vi "getEventID.vi"(8 "error in (no error)":errorcluster, 11 "IEventPacket in":refnum<class "IEventPacket.lvclass">) -> (0 "error out":errorcluster, 2 "EventID out":string, 3 "IEventPacket out":refnum<class "IEventPacket.lvclass">)   [LabVIEW 2022 SP3, in "openDAQ.lvlib" / "IBaseObject.lvlib" / "IPacket.lvlib" / "IEventPacket.lvlib" / "IEventPacket.lvclass"]
uses:
  <instrlib>/openDAQ/Public/Classes/IEventPacket/IEventPacket.lvclass
  C:/Program Files (x86)/National Instruments/LabVIEW 2022/instr.lib/openDAQ/Public/Classes/IBaseObject/IBaseObject.lvclass
  <instrlib>/openDAQ/Public/Classes/IBaseObject/IBaseObject.lvclass/IBaseObject.ctl
  <instrlib>/openDAQ/Public/Classes/IBaseObject/Accessor/Read reference.vi
  <instrlib>/openDAQ/Public/Classes/IBaseObject/Accessor/Write reference.vi
  <instrlib>/openDAQ/Public/Classes/daqCoreTypes/IString/IString.lvclass
  <instrlib>/openDAQ/Binaries/Windows/x86/copendaq32.dll
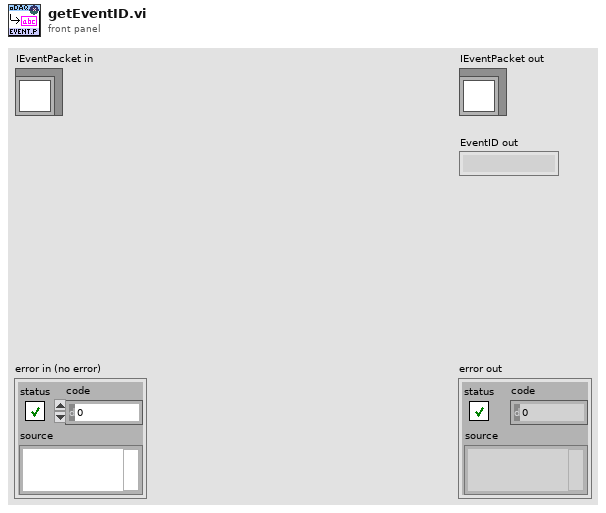
[diagram p1: front panel]
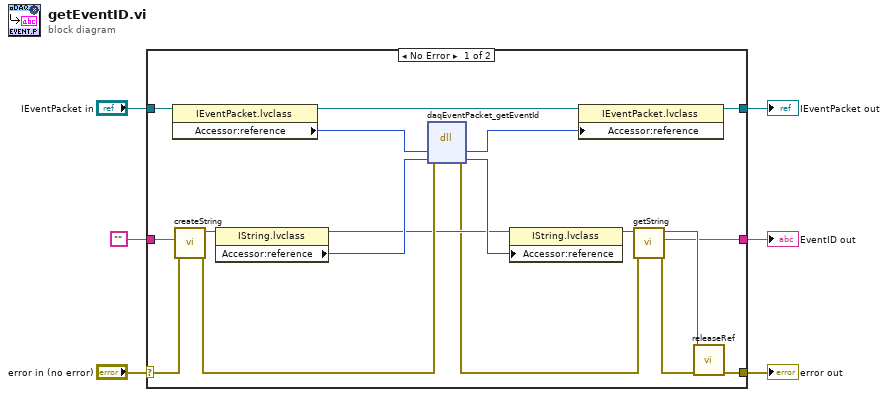
[diagram p0: block diagram]
diagram:
  n1 = case shown="No Error" "error in (no error)" {
    selector: "error in (no error)" -> [w21 w27]
    tunnel: [w12 w27] -> w5
    tunnel: [w7 w26] -> w3
    tunnel: "IEventPacket in" -> [w24 w26]
    tunnel: [w10 w25] -> w1
    tunnel: "" -> [w9 w25]
    frame No Error {
      n2 = property class="IEventPacket.lvclass"(reference=w24) -> (reference out=w8:refnum<class "IEventPacket.lvclass">, "Accessor:reference"=w23:i64)  [unwired: 1 in, 1 out]
      n3 = call <instrlib>:"createString.vi"("error in (no error)"=w21, "String"=w9) -> ("error out"=w20:errorcluster, "IString out"=w19:refnum<class "IString.lvclass">)  [unwired: 8 in]
      n4 = property class="IString.lvclass"(reference=w19) -> (reference out=w16:refnum<class "IString.lvclass">, "Accessor:reference"=w18:i64)  [unwired: 1 in, 1 out]
      n5 = dll-call lib="C:/Program Files (x86)/National Instruments/LabVIEW 2022/instr.lib/openDAQ/Binaries/Windows/x86/copendaq*.*" fn="daqEventPacket_getEventId"(error in=w20, "eventPacket"=w23, "eventId"=w18) -> (error out=w14:errorcluster, "eventPacket"=w22:i64, "eventId"=w17:i64)  [unwired: 3 in, 1 out]
      n6 = property class="IString.lvclass"(reference=w16, "Accessor:reference"=w17) -> (reference out=w15:refnum<class "IString.lvclass">)  [unwired: 1 in, 1 out]
      n7 = property class="IEventPacket.lvclass"(reference=w8, "Accessor:reference"=w22) -> (reference out=w7:refnum<class "IEventPacket.lvclass">)  [unwired: 1 in, 1 out]
      n8 = call <instrlib>:"getString.vi"("error in (no error)"=w14, "IString in"=w15) -> ("error out"=w13:errorcluster, "String out"=w10:string, "IString out"=w11:refnum<class "IString.lvclass">)  [unwired: 7 in]
      n9 = call-dynamic "releaseRef.vi"("error in (no error)"=w13, "IBaseObject in"=w11) -> ("error out"=w12:errorcluster)  [unwired: 9 in]
    }
    frame Error {
    }
  }
  "error out" <- w5
  "IEventPacket out" <- w3
  "EventID out" <- w1
